vi "Get Pulse State.vi"(8 "error in (no error)":errorcluster, 11 "Micron sm Digitizer in":refnum<class "Micron sm Digitizer.lvclass">) -> (0 "error out":errorcluster, 1 "Result ready":bool, 2 "Armed":bool, 3 "Micron sm Digitizer out":refnum<class "Micron sm Digitizer.lvclass">, 4 "Recording compleste":bool)   [LabVIEW 2024, in "Micron sm Digitizer.lvclass"]
uses:
  Micron sm Digitizer.lvclass
  Micron sm Digitizer.lvclass/Micron sm Digitizer.ctl
  Micron Optics sm130/Micron Optics sm130.lvlib
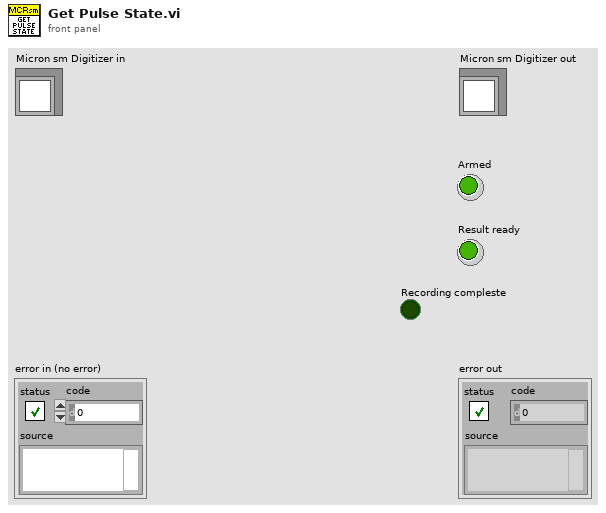
[diagram p1: front panel]
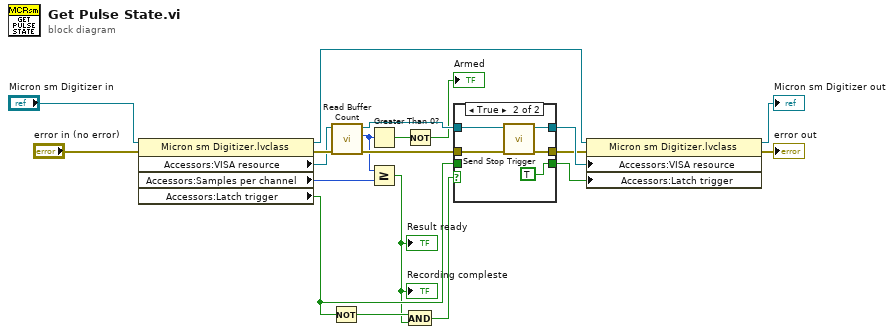
[diagram p0: block diagram]
diagram:
  n1 = property class="Micron sm Digitizer.lvclass"(reference="Micron sm Digitizer in", error in="error in (no error)") -> (reference out=w7:refnum<class "Micron sm Digitizer.lvclass">, error out=w9:errorcluster, "Accessors:VISA resource"=w8:refnum<visa-resource-name>, "Accessors:Samples per channel"=w12:i32, "Accessors:Latch trigger"=w19:bool)
  n2 = Not(x=w19) -> (.not. x?=w18:bool)
  n3 = call "Read Buffer Count.vi"("error in"=w9, "VISA resource name"=w8) -> ("error out"=w13:errorcluster, "count"=w11:i32, "VISA resource name out"=w15:refnum<visa-resource-name>)  [unwired: 6 in, 1 out]
  n4 = Greater Than 0?(x=w11) -> (x > 0?=w10:bool)
  n5 = Greater Or Equal?(x=w11, y=w12) -> (x >= y?=w1:bool)
  "Result ready" <- w1
  "Recording compleste" <- w1
  n6 = Not(x=w10) -> (.not. x?=→"Armed":bool)
  n7 = And(x=w18, y=w1) -> (x .and. y?=w17:bool)
  n8 = case shown="True" w17 {
    tunnel: w13 -> [w22 w28]
    tunnel: [w22 w27] -> w14
    tunnel: w15 -> [w23 w26]
    tunnel: [w23 w25] -> w16
    tunnel: w19 -> [w21 _]
    tunnel: [w21 TRUE ("Accessors:Latch trigger")] -> w20
    frame False {
    }
    frame True {
      n9 = call "Send Stop Trigger.vi"("error in (no error)"=w28, "VISA resource name"=w26) -> ("error out"=w27:errorcluster, "VISA resource name out"=w25:refnum<visa-resource-name>)  [unwired: 8 in]
    }
  }
  n10 = property class="Micron sm Digitizer.lvclass"(reference=w7, error in=w14, "Accessors:VISA resource"=w16, "Accessors:Latch trigger"=w20) -> (reference out=→"Micron sm Digitizer out":refnum<class "Micron sm Digitizer.lvclass">, error out=→"error out":errorcluster)
